vi "xeva-getParam.vi"(2 "error in (no error)":errorcluster, 3 "xeva-camref":T2) -> (0 "error out":errorcluster, 1 "xeva-parameters":T1 {"time" format="%#.2f"})   [LabVIEW 2017]
uses:
  <vilib>/Xenics Infrared Solutions/Xeneth LabVIEW API/VIs/Controls/Camara.ctl
  <vilib>/Xenics Infrared Solutions/Xeneth LabVIEW API/Xeneth.lvlib
panel:
  out "status array":bool[](array[boolean])
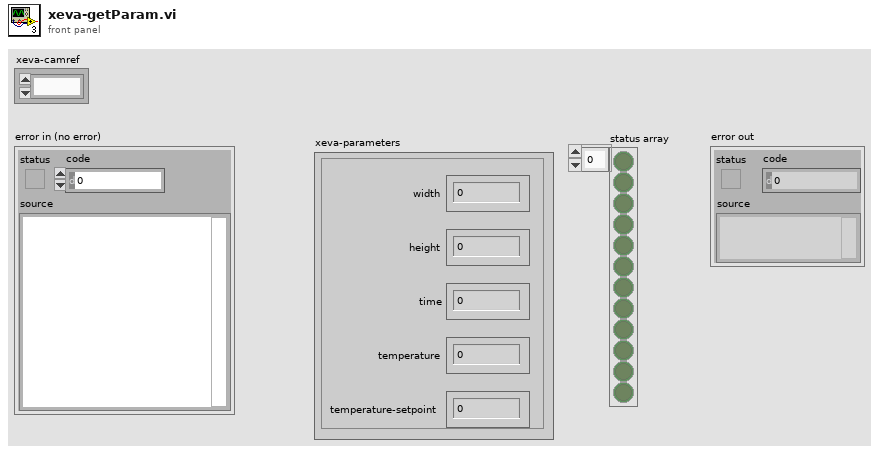
[diagram p1: front panel]
types:
  T1 = cluster{"width":u32, "height":u32, "time":dbl, "temperature":dbl, "temperature-setpoint":dbl}
  T2 = typedef "Xeneth.lvlib/Camara.ctl" = refnum<k1>
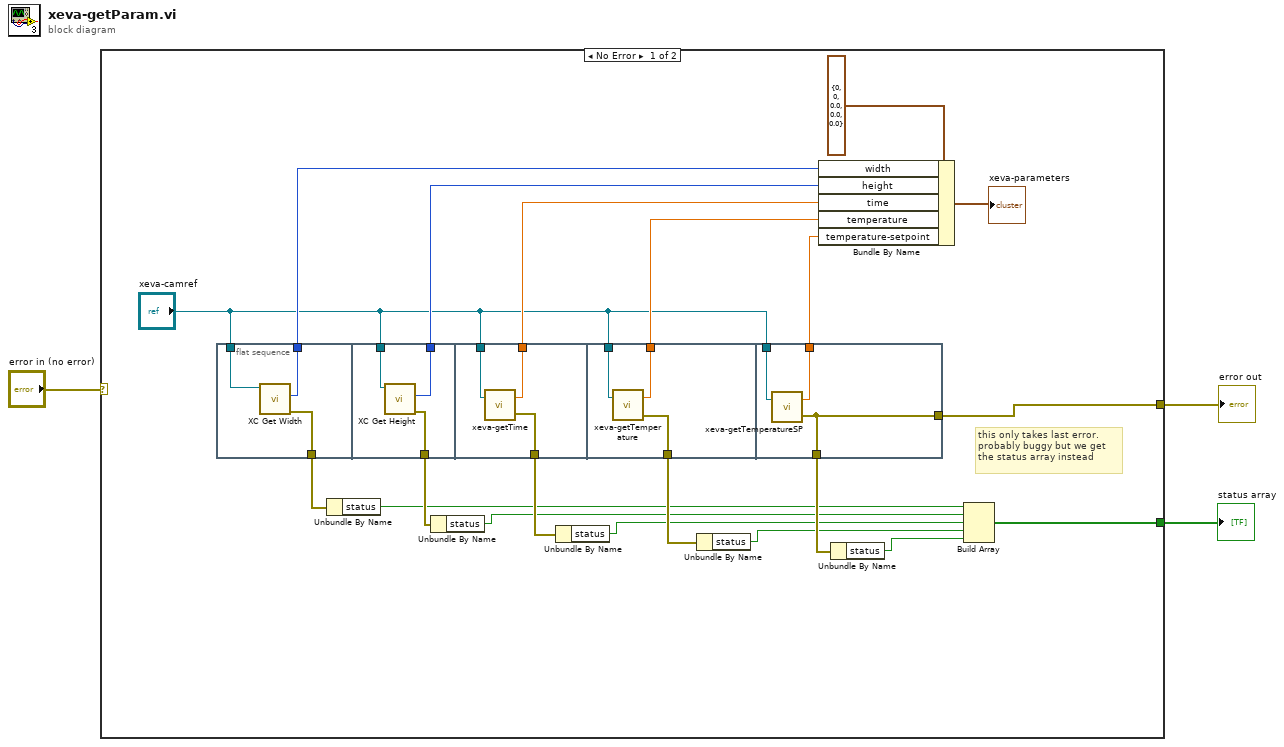
[diagram p0: block diagram]
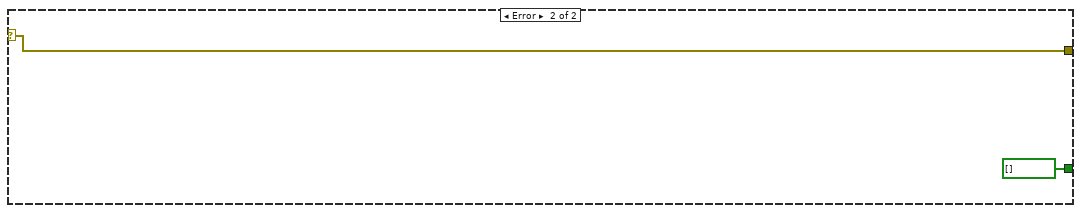
[diagram p2: hidden frame]
diagram:
  n1 = case shown="No Error" "error in (no error)" {
    selector: "error in (no error)" -> [_ w40]
    tunnel: [w10 w40] -> w2
    tunnel: [w4 bool[] []] -> w1
    frame No Error {
      # "this only takes last error.\nprobably buggy but we get\nthe status array instead"
      n2 = flat-sequence {
        tunnel: [w26] -> w23
        tunnel: "xeva-camref" -> [w25]
        tunnel: [w24] -> w15
        tunnel: "xeva-camref" -> [w29]
        tunnel: [w28] -> w20
        tunnel: [w27] -> w14
        tunnel: "xeva-camref" -> [w32]
        tunnel: [w31] -> w19
        tunnel: [w30] -> w13
        tunnel: "xeva-camref" -> [w35]
        tunnel: [w34] -> w18
        tunnel: [w33] -> w12
        tunnel: "xeva-camref" -> [w38]
        tunnel: [w37] -> w16
        tunnel: [w36] -> w10
        tunnel: [w36] -> w11
        frame #0 {
          n3 = call <vilib>:"XC Get Width.vi"("Cam Ref"=w25) -> ("error out"=w24:errorcluster, "Width"=w26:u32)  [unwired: 8 in, 1 out]
        }
        frame #1 {
          n4 = call <vilib>:"XC Get Height.vi"("Cam Ref"=w29) -> ("error out"=w27:errorcluster, "Height"=w28:u32)  [unwired: 8 in, 1 out]
        }
        frame #2 {
          n5 = call "xeva-getTime.vi"("xeva-camref"=w32) -> ("error out"=w30:errorcluster, "xeva-time"=w31:dbl)  [unwired: 1 in]
        }
        frame #3 {
          n6 = call "xeva-getTemperature.vi"("xeva-camref"=w35) -> ("error out"=w33:errorcluster, "xeva-temperature"=w34:dbl)  [unwired: 1 in]
        }
        frame #4 {
          n7 = call "xeva-getTemperatureSP.vi"("xeva-camref"=w38) -> ("error out"=w36:errorcluster, "xeva-temperature-setpoint"=w37:dbl)  [unwired: 1 in]
        }
      }
      n8 = Unbundle By Name(w15) -> ("status"=w9:bool)
      n9 = Unbundle By Name(w14) -> ("status"=w8:bool)
      n10 = Unbundle By Name(w13) -> ("status"=w7:bool)
      n11 = Unbundle By Name(w12) -> ("status"=w6:bool)
      n12 = Bundle By Name(cluster=T1 {"width"=0, "height"=0, "time"=0.0, "temperature"=0.0, "temperature-setpoint"=0.0} ("xeneth-parameters"), "width"=w23, "height"=w20, "time"=w19, "temperature"=w18, "temperature-setpoint"=w16) -> (→"xeva-parameters":T1)
      n13 = Unbundle By Name(w11) -> ("status"=w5:bool)
      n14 = Build Array(w9, w8, w7, w6, w5) -> (w4:bool[])
    }
    frame Error {
    }
  }
  "error out" <- w2
  "status array" <- w1
